vi "甩线新增两点补偿.vi"(9 "进出线选项":T1, 10 "布尔":bool, 11 "数组输入":string[](array[string])) -> (3 "数组输出":string[](array[string]))   [LabVIEW 2014]
uses:
  Global.vi
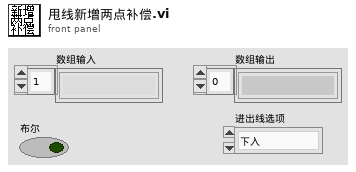
[diagram p1: front panel]
types:
  T1 = typedef "进出线选项.ctl" = enum16{"下入", "上入", "下出", "上出"}
  T2 = typedef "XYPos.ctl" = cluster{"X":dbl, "Y":dbl}
  T3 = typedef "mark规格.ctl" = cluster{"X下限":dbl, "X上限":dbl, "Y下限":dbl, "Y 上限":dbl, "angle下限":dbl, "angle上限":dbl}
  T4 = cluster{"甩线补偿值":cluster{"下边":dbl, "距离上边":dbl, "左边":dbl, "右边":dbl}, "补偿甩线坐标偏移":T2, "mark点模组补偿":T2, "出线补偿值":dbl, "mark规格":T3}
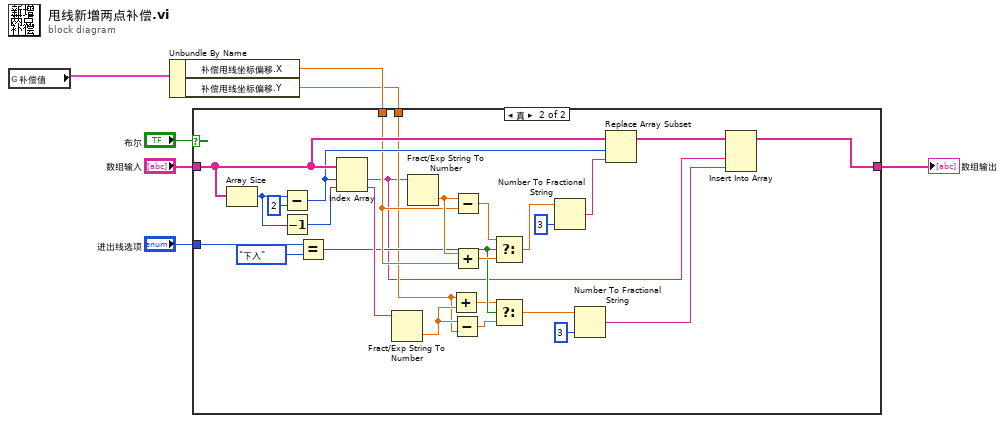
[diagram p0: block diagram]
diagram:
  n1 = global read "Global.vi" "补偿值"() -> (w1:T4)
  n2 = Unbundle By Name(w1) -> ("补偿甩线坐标偏移.X"=w3:dbl, "补偿甩线坐标偏移.Y"=w2:dbl)
  n3 = case shown="真" "布尔" {
    tunnel: "数组输入" -> [w8 w30]
    tunnel: [w8 w21] -> w7
    tunnel: "进出线选项" -> [_ w32]
    tunnel: w3 -> [_ w24]
    tunnel: w2 -> [_ w14]
    frame False {
    }
    frame True {
      n4 = Array Size(array=w30) -> (size(s)=w20:i32)
      n5 = Subtract(x=w20, y=2) -> (x-y=w29:i32)
      n6 = Decrement(x=w20) -> (x-1=w19:i32)
      n7 = Equal?(x=w32, y=进出线选项."下入") -> (x = y?=w17:bool)
      n8 = Index Array(array=w30, index #1=w29, index #2=w19) -> (element #1=w12:string, element #2=w18:string)
      n9 = Fract/Exp String To Number(string=w18) -> (number=w15:dbl)  [unwired: 3 in, 1 out]
      n10 = Fract/Exp String To Number(string=w12) -> (number=w25:dbl)  [unwired: 3 in, 1 out]
      n11 = Add(x=w14, y=w15) -> (x+y=w16:dbl)
      n12 = Subtract(x=w15, y=w14) -> (x-y=w13:dbl)
      n13 = Subtract(x=w25, y=w24) -> (x-y=w27:dbl)
      n14 = Add(x=w25, y=w24) -> (x+y=w23:dbl)
      n15 = Select(t=w27, s=w17, f=w23) -> (s? t:f=w26:dbl)
      n16 = Select(t=w16, s=w17, f=w13) -> (s? t:f=w10:dbl)
      n17 = Number To Fractional String(number=w26, precision (6)=i16 3 ("精度(6)")) -> (F-format string=w28:string)  [unwired: 2 in]
      n18 = Number To Fractional String(number=w10, precision (6)=i16 3 ("精度(6)")) -> (F-format string=w9:string)  [unwired: 2 in]
      n19 = Replace Array Subset(array=w30, new element=w28, index=w29) -> (w22:string[])
      n20 = Insert Into Array(array=w22, new element #1=w12, new element #2=w9) -> (w21:string[])  [unwired: 1 in]
    }
  }
  "数组输出" <- w7
